vi "Scatter-Gather Test.vi"() -> ()   [LabVIEW 2016]
uses:
  Source/GE 5565PIORC/Controls/Interrupt Enables.ctl
  Source/GE 5565PIORC/GE 5565PIORC.lvclass/GE 5565PIORC.ctl
  Source/GE 5565PIORC/VIs/DMA/DMA.Write (Scatter-Gather).vi
  Source/GE 5565PIORC/VIs/DMA/DMA.Configure.vi
  Source/GE 5565PIORC/VIs/DMA/DMA.Configure (Scatter-Gather).vi
  Source/GE 5565PIORC/VIs/DMA/DMA.Start Transfer.vi
  Source/GE 5565PIORC/VIs/DMA/DMA.Wait for Done Interrupt Event.vi
  Source/GE 5565PIORC/VIs/Interrupts/Discard PXI Interrupt Events.vi
  Source/GE 5565PIORC/VIs/Interrupts/Wait for PXI Interrupt Events.vi
  <vilib>/Utility/error.llb/Clear Errors.vi
  Source/GE 5565PIORC/VIs/Block Operations/Allocate Multiple Blocks.vi
  Source/GE 5565PIORC/VIs/DMA/Scatter-Gather/DMA.Scatter-Gather.Get Transfer Size.vi
  Source/GE 5565PIORC/VIs/Registers/Local Configuration.DMAMODE0.Scatter-Gather Enable.Set.vi
  Source/GE 5565PIORC/VIs/Registers/Local Configuration.DMADPR0.First Descriptor Address.Set.vi
  Source/GE 5565PIORC/VIs/Registers/Local Configuration.Local Address.Set.vi
  Source/GE 5565PIORC/VIs/Registers/Local Configuration.Transfer Size.Set.vi
  Source/GE 5565PIORC/VIs/Registers/Local Configuration.DMADPR0.Transfer Direction.Set.vi
  Source/GE 5565PIORC/VIs/Registers/Local Configuration.DMACSR0.DMA Start.Set.vi
  Source/GE 5565PIORC/VIs/Registers/Local Configuration.DMACSR0.DMA Clear Interrupt.Set.vi
  Source/GE 5565PIORC/GE 5565PIORC.lvclass
panel:
  out "66 MHz Capable?":bool
  out "Latency (cycles)":u8
  out "Transfer Size (bytes)":u32
  out "us period 2":u32
  out "Data in":dbl[](array[numeric])
  out "us period":u32
  in  "stop":bool
  in  "RFM Address":u32 format="%08x"
  out "Block 3":dbl[](array[numeric])
  out "Block 2":dbl[](array[numeric])
  in  "samples":i32=10000
  out "Block 1":dbl[](array[numeric])
  out "error out":errorcluster
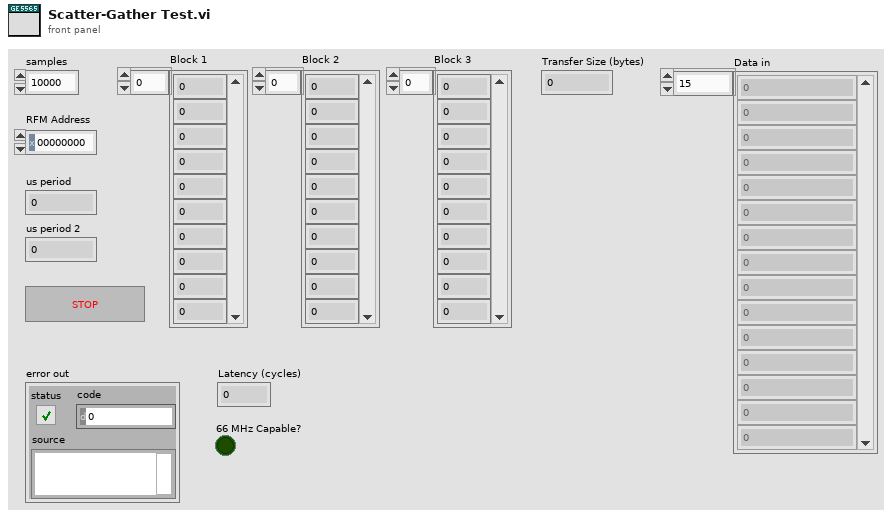
[diagram p1: front panel]
types:
  T1 = typedef "GE 5565PIORC.lvclass/Interrupt Enables.ctl" = cluster{"PCI Interrupt":bool, "Local Interrupt":bool, "DMA Interrupt":bool}
  T2 = typedef "GE 5565PIORC.lvclass/DMA Block Descriptor.ctl" = cluster{"descriptor ptr (VISA)":u32, "descriptor size":u32, "descriptor ptr (aligned)":u32, "data ptr (lower)":u32, "data ptr (upper)":u32, "data size":u32, "next descriptor ptr":u32}
  T3 = typedef "GE 5565PIORC.lvclass/DMA Transfer Spec (Scatter-Gather).ctl" = cluster{"RFM Address":u32, "Block Descriptors":T2[]}
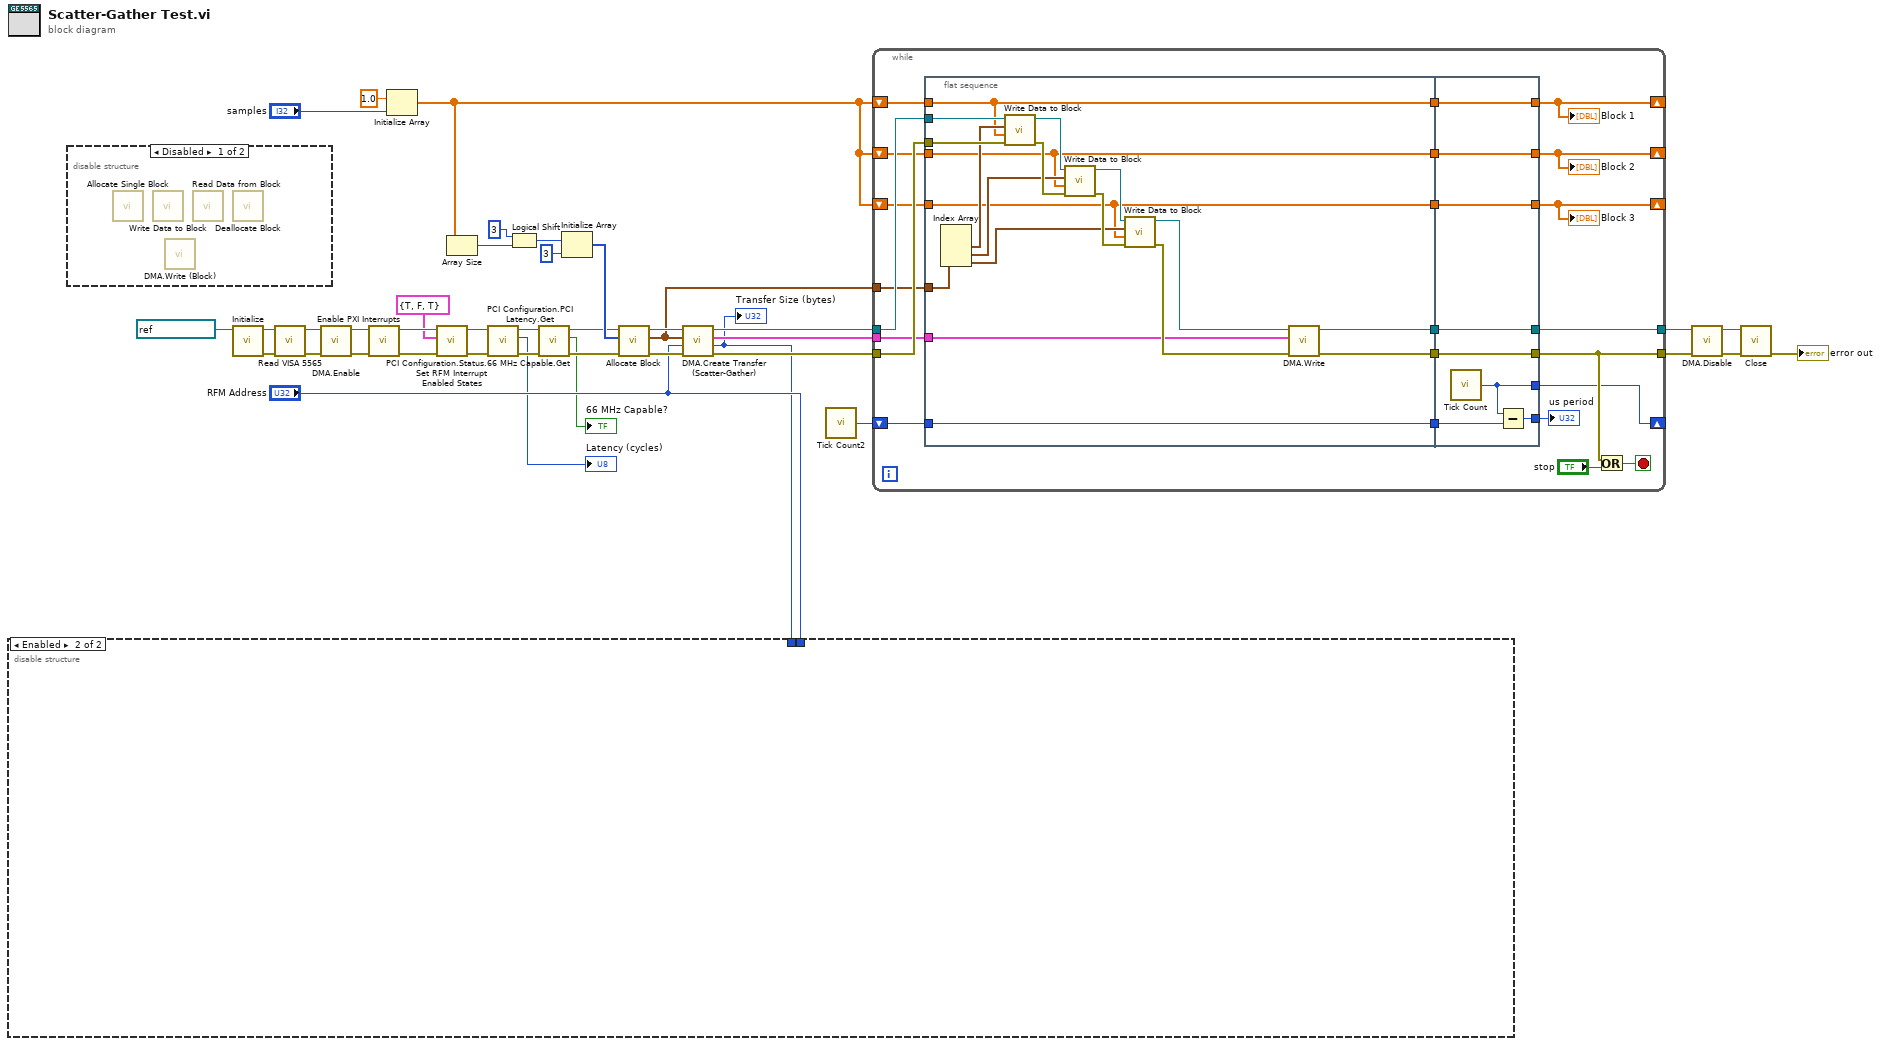
[diagram p0: block diagram]
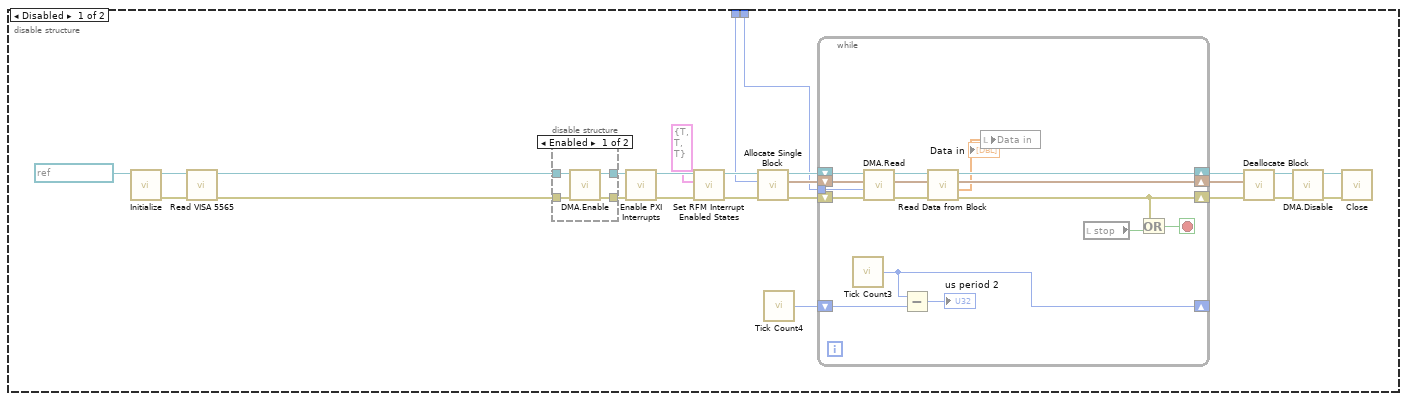
[diagram p2: hidden frame]
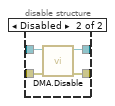
[diagram p3: hidden frame]
diagram:
  n1 = disable-structure shown="Disabled" {
    frame Disabled {
      n2 = call "Allocate Single Block.vi"() -> ()  [unwired: 9 in, 3 out]
      n3 = call "Write Data to Block.vi"() -> ()  [unwired: 9 in, 3 out]
      n4 = call "DMA.Write (Block).vi"() -> ()  [unwired: 9 in, 3 out]
      n5 = call "Read Data from Block.vi"() -> ()  [unwired: 8 in, 4 out]
      n6 = call "Deallocate Block.vi"() -> ()  [unwired: 10 in, 2 out]
    }
    frame Enabled {
    }
  }
  n7 = call "Initialize.vi"("VISA resource name"=refnum<visa-resource-name> "RefMem2") -> ("error out"=w20:errorcluster, "GE 5565PIORC"=w21:refnum<class "GE 5565PIORC.lvclass">)  [unwired: 9 in]
  n8 = call "Read VISA 5565.vi"("error in (no error)"=w20, "GE 5565PIORC in"=w21) -> ("error out"=w18:errorcluster, "GE 5565PIORC out"=w19:refnum<class "GE 5565PIORC.lvclass">)  [unwired: 7 in, 1 out]
  n9 = call "DMA.Enable.vi"("error in (no error)"=w18, "GE 5565PIORC in"=w19) -> ("error out"=w39:errorcluster, "GE 5565PIORC out"=w17:refnum<class "GE 5565PIORC.lvclass">)  [unwired: 8 in]
  n10 = call "Enable PXI Interrupts.vi"("error in (no error)"=w39, "GE 5565PIORC in"=w17) -> ("error out"=w37:errorcluster, "GE 5565PIORC out"=w38:refnum<class "GE 5565PIORC.lvclass">)  [unwired: 8 in]
  n11 = Initialize Array(1.0 ("element"), "samples") -> (w31:dbl[])
  n12 = call "Set RFM Interrupt Enabled States.vi"("error in (no error)"=w37, "Interrupt Enables"=T1 {"PCI Interrupt"=TRUE, "Local Interrupt"=FALSE, "DMA Interrupt"=TRUE}, "GE 5565PIORC in"=w38) -> ("error out"=w7:errorcluster, "GE 5565PIORC out"=w8:refnum<class "GE 5565PIORC.lvclass">)  [unwired: 7 in]
  n13 = Array Size(array=w31) -> (size(s)=w33:i32)
  n14 = call "PCI Configuration.PCI Latency.Get.vi"("error in (no error)"=w7, "GE 5565PIORC"=w8) -> ("error out"=w5:errorcluster, "Latency (cycles)"=→"Latency (cycles)":u8, "GE 5565PIORC out"=w6:refnum<class "GE 5565PIORC.lvclass">)  [unwired: 7 in]
  n15 = Logical Shift(y=i16 3, x=w33) -> (x << y=w24:i32)
  n16 = call "PCI Configuration.Status.66 MHz Capable.Get.vi"("error in (no error)"=w5, "GE 5565PIORC"=w6) -> ("error out"=w2:errorcluster, "66 MHz Capable?"=→"66 MHz Capable?":bool, "GE 5565PIORC out"=w4:refnum<class "GE 5565PIORC.lvclass">)  [unwired: 7 in]
  n17 = Initialize Array(w24, 3 ("dimension size")) -> (w22:i32[])
  n18 = call-poly "Allocate Block.vi"("error in (no error)"=w2, "sizes (bytes)"=w22, "GE 5565PIORC in"=w4) -> ("error out"=w14:errorcluster, "Block Descriptors"=w12:T2[], "GE 5565PIORC out"=w16:refnum<class "GE 5565PIORC.lvclass">)  [unwired: 6 in]
  n19 = call "DMA.Create Transfer (Scatter-Gather).vi"("error in (no error)"=w14, "RFM Offset"="RFM Address", "Block Descriptors"=w12, "GE 5565PIORC in"=w16) -> ("error out"=w13:errorcluster, "Transfer Size (bytes)"=w9:u32, "Scatter-Gather Transfer Spec"=w10:T3, "GE 5565PIORC out"=w15:refnum<class "GE 5565PIORC.lvclass">)  [unwired: 4 in]
  "Transfer Size (bytes)" <- w9
  n20 = disable-structure shown="Enabled" {
    disable-tunnel: "RFM Address" -> [w42 _]
    disable-tunnel: w9 -> [w41 _]
    frame Disabled {
      n21 = call "Initialize.vi"("VISA resource name"=refnum<visa-resource-name> "RefMem1") -> ("error out"=w44:errorcluster, "GE 5565PIORC"=w46:refnum<class "GE 5565PIORC.lvclass">)  [unwired: 9 in]
      n22 = call "Read VISA 5565.vi"("error in (no error)"=w44, "GE 5565PIORC in"=w46) -> ("error out"=w43:errorcluster, "GE 5565PIORC out"=w45:refnum<class "GE 5565PIORC.lvclass">)  [unwired: 7 in, 1 out]
      n23 = disable-structure shown="Enabled" {
        disable-tunnel: w43 -> [w69 w72]
        disable-tunnel: [w68 w71] -> w64
        disable-tunnel: [w67 w70] -> w63
        disable-tunnel: w45 -> [w66 w73]
        frame Enabled {
          n24 = call "DMA.Enable.vi"("error in (no error)"=w69, "GE 5565PIORC in"=w66) -> ("error out"=w67:errorcluster, "GE 5565PIORC out"=w68:refnum<class "GE 5565PIORC.lvclass">)  [unwired: 8 in]
        }
        frame Disabled {
          n25 = call "DMA.Disable.vi"("error in (no error)"=w72, "GE 5565PIORC in"=w73) -> ("error out"=w70:errorcluster, "GE 5565PIORC out"=w71:refnum<class "GE 5565PIORC.lvclass">)  [unwired: 8 in]
        }
      }
      n26 = call "Enable PXI Interrupts.vi"("error in (no error)"=w63, "GE 5565PIORC in"=w64) -> ("error out"=w61:errorcluster, "GE 5565PIORC out"=w62:refnum<class "GE 5565PIORC.lvclass">)  [unwired: 8 in]
      n27 = call "Set RFM Interrupt Enabled States.vi"("error in (no error)"=w61, "Interrupt Enables"=T1 {"PCI Interrupt"=TRUE, "Local Interrupt"=TRUE, "DMA Interrupt"=TRUE}, "GE 5565PIORC in"=w62) -> ("error out"=w59:errorcluster, "GE 5565PIORC out"=w60:refnum<class "GE 5565PIORC.lvclass">)  [unwired: 7 in]
      n28 = call "Allocate Single Block.vi"("error in (no error)"=w59, "size (bytes)"=w41, "GE 5565PIORC in"=w60) -> ("error out"=w53:errorcluster, "Block Descriptor"=w52:T2, "GE 5565PIORC out"=w54:refnum<class "GE 5565PIORC.lvclass">)  [unwired: 6 in]
      n29 = call "Tick Count4"() -> ("Tick Count(uSec)"=w47:u32)
      n30 = while {
        shift-right: [w78] -> w57
        shift-left: w54 -> [w85]
        shift-right: [w76] -> w55
        shift-left: w53 -> [w84]
        shift-right: [w77] -> w56
        shift-left: w52 -> [w83]
        shift-right: [w86] -> _
        shift-left: w47 -> [w88]
        tunnel: w42 -> [w82]
        stop <- w89 stop-if-true
        n31 = call "Tick Count3"() -> ("Tick Count(uSec)"=w86:u32)
        n32 = call "DMA.Read.vi"("error in (no error)"=w84, "RFM Address"=w82, "Block Descriptor"=w83, "GE 5565PIORC"=w85) -> ("error out"=w81:errorcluster, "Block Descriptor out"=w79:T2, "GE 5565PIORC out"=w80:refnum<class "GE 5565PIORC.lvclass">)  [unwired: 4 in, 1 out]
        n33 = Subtract(x=w86, y=w88) -> (x-y=→"us period 2":u32)
        n34 = call "Read Data from Block.vi"("error in (no error)"=w81, "Block Descriptor"=w79, "GE 5565PIORC"=w80) -> ("error out"=w76:errorcluster, "Data"=w75:dbl[], "Block Descriptor out"=w77:T2, "GE 5565PIORC out"=w78:refnum<class "GE 5565PIORC.lvclass">)  [unwired: 5 in]
        n35 = local write "Data in"(w75) -> ()
        n36 = local read "stop"() -> (w74:bool)
        n37 = Or(x=w76, y=w74) -> (x .or. y?=w89:bool)
      }
      n38 = call "Deallocate Block.vi"("error in (no error)"=w55, "Block Descriptor"=w56, "GE 5565PIORC in"=w57) -> ("error out"=w50:errorcluster, "GE 5565PIORC out"=w51:refnum<class "GE 5565PIORC.lvclass">)  [unwired: 7 in]
      n39 = call "DMA.Disable.vi"("error in (no error)"=w50, "GE 5565PIORC in"=w51) -> ("error out"=w48:errorcluster, "GE 5565PIORC out"=w49:refnum<class "GE 5565PIORC.lvclass">)  [unwired: 8 in]
      n40 = call "Close.vi"("error in (no error)"=w48, "GE 5565PIORC in"=w49) -> ()  [unwired: 9 in, 1 out]
    }
    frame Enabled {
    }
  }
  n41 = call "Tick Count2"() -> ("Tick Count(uSec)"=w25:u32)
  n42 = while {
    shift-right: [w103] -> _
    shift-left: w31 -> [w109]
    shift-right: [w102] -> _
    shift-left: w31 -> [w108]
    shift-right: [w101] -> _
    shift-left: w31 -> [w107]
    tunnel: w15 -> [w112]
    tunnel: w13 -> [w111]
    tunnel: [w110] -> w28
    tunnel: [w105] -> w27
    shift-right: [w93] -> _
    shift-left: w25 -> [w95]
    tunnel: w12 -> [w91]
    tunnel: w10 -> [w90]
    stop <- w104 stop-if-true
    n43 = flat-sequence {
      tunnel: w112 -> [w131]
      tunnel: w111 -> [w130]
      tunnel: w109 -> [w122]
      tunnel: w108 -> [w121]
      tunnel: w107 -> [w120]
      tunnel: [w116] -> w100
      tunnel: [w114] -> w99
      tunnel: [w122] -> w98
      tunnel: [w121] -> w97
      tunnel: [w120] -> w96
      tunnel: w95 -> [w119]
      tunnel: [w119] -> w94
      tunnel: w91 -> [w118]
      tunnel: w90 -> [w113]
      tunnel: [w135] -> w101
      tunnel: [w136] -> w102
      tunnel: [w137] -> w103
      tunnel: [w138] -> w105
      tunnel: [w139] -> w110
      tunnel: w100 -> [w139]
      tunnel: w99 -> [w138]
      tunnel: w98 -> [w137]
      tunnel: w97 -> [w136]
      tunnel: w96 -> [w135]
      tunnel: w94 -> [w134]
      tunnel: [w133] -> w93
      tunnel: [w132] -> w92
      frame #0 {
        n44 = Index Array(array=w118) -> (element #1=w123:T2, element #2=w124:T2, element #3=w125:T2)  [unwired: 3 in]
        n45 = call "Write Data to Block.vi"("error in (no error)"=w130, "Data"=w122, "Block Descriptor"=w123, "GE 5565PIORC"=w131) -> ("error out"=w127:errorcluster, "GE 5565PIORC out"=w129:refnum<class "GE 5565PIORC.lvclass">)  [unwired: 5 in, 1 out]
        n46 = call "Write Data to Block.vi"("error in (no error)"=w127, "Data"=w121, "Block Descriptor"=w124, "GE 5565PIORC"=w129) -> ("error out"=w126:errorcluster, "GE 5565PIORC out"=w128:refnum<class "GE 5565PIORC.lvclass">)  [unwired: 5 in, 1 out]
        n47 = call "Write Data to Block.vi"("error in (no error)"=w126, "Data"=w120, "Block Descriptor"=w125, "GE 5565PIORC"=w128) -> ("error out"=w115:errorcluster, "GE 5565PIORC out"=w117:refnum<class "GE 5565PIORC.lvclass">)  [unwired: 5 in, 1 out]
        n48 = call-poly "DMA.Write.vi"("error in (no error)"=w115, "Scatter-Gather Transfer Spec"=w113, "GE 5565PIORC"=w117) -> ("error out"=w114:errorcluster, "GE 5565PIORC out"=w116:refnum<class "GE 5565PIORC.lvclass">)  [unwired: 6 in, 1 out]
      }
      frame #1 {
        n49 = call "Tick Count"() -> ("Tick Count(uSec)"=w133:u32)
        n50 = Subtract(x=w133, y=w134) -> (x-y=w132:u32)
      }
    }
    n51 = Or(x=w105, y="stop") -> (x .or. y?=w104:bool)
    "Block 1" <- w103
    "Block 2" <- w102
    "Block 3" <- w101
    "us period" <- w92
  }
  n52 = call "DMA.Disable.vi"("error in (no error)"=w27, "GE 5565PIORC in"=w28) -> ("error out"=w29:errorcluster, "GE 5565PIORC out"=w30:refnum<class "GE 5565PIORC.lvclass">)  [unwired: 8 in]
  n53 = call "Close.vi"("error in (no error)"=w29, "GE 5565PIORC in"=w30) -> ("error out"=→"error out":errorcluster)  [unwired: 9 in]
